vi "Finish.vi"(8 "error in (no error)":errorcluster, 11 "Dev Grabber in":refnum<class "Dev Grabber.lvclass">) -> (0 "error out":errorcluster, 3 "Dev Grabber out":refnum<class "Dev Grabber.lvclass">)   [LabVIEW 2014, in "Dev Grabber.lvlib" / "Dev Grabber.lvclass"]
uses:
  Dev Grabber.lvclass
  Dev Grabber.lvclass/Dev Grabber.ctl
  Robot/Grabber/Grabber Class/Grabber.lvclass
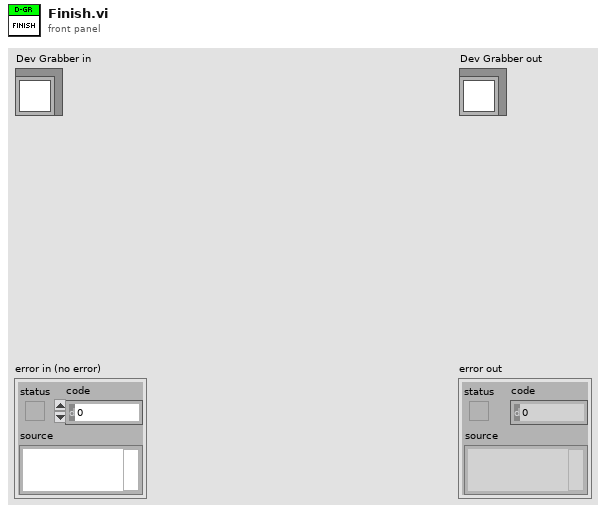
[diagram p1: front panel]
types:
  T1 = typedef "WPI_SolenoidDevRef.ctl" = cluster{"DevStatus":errorcluster, "Pneumatics Control Module":u8, "Forward Solenoid Channel":T2, "Reverse Solenoid Channel":T2}
  T2 = typedef "WPI_SolenoidChannel.ctl" = enum8{"Solenoid 0", "Solenoid 1", "Solenoid 2", "Solenoid 3", "Solenoid 4", "Solenoid 5", "Solenoid 6", "Solenoid 7", "Invalid"}
  T3 = typedef "WPI_MotorControlDeviceRef.ctl" = cluster{"DeviceStatus":errorcluster, "Type":T4, "PWM":cluster{"Controller":T5, "PWM Channel":T6, "DeadBand":T7}, "CAN":cluster{"Device Number":u8, "Control Mode":T8, "Semaphore":T9, "Max Vout":dbl, "TalonSRX Control Mode":T10}, "Invert":bool, "TransformRef":T11, "InvTransformRef":T11}
  T4 = typedef "WPI_MotorControlType.ctl" = enum16{"PWM", "CAN", "CANTalonSRX"}
  T5 = typedef "FPGA_TypedefDigitalModule.ctl" = enum16{"Controller 1"}
  T6 = typedef "FPGA_DIOPWMChannel.ctl" = enum8{"PWM 0", "PWM 1", "PWM 2", "PWM 3", "PWM 4", "PWM 5", "PWM 6", "PWM 7", "PWM 8", "PWM 9", "PWM MXP 0", "PWM MXP 1", "PWM MXP 2", "PWM MXP 3", "PWM MXP 4", "PWM MXP 5", "PWM MXP 6", "PWM MXP 7", "PWM MXP 8", "PWM MXP 9", "Invalid"}
  T7 = typedef "WPI_PWMDeadband.ctl" = cluster{"Name":string, "maxPositivePwm":i32, "minPositivePwm":i32, "centerPwm":i32, "maxNegativePwm":i32, "minNegativePwm":i32, "angularRange":u16}
  T8 = typedef "WPI_CANJaguar_ControlMode.ctl" = enum8{"Percent VBus", "Current", "Speed", "Position", "Voltage"}
  T9 = typedef "Semaphore RefNum" = refnum<k1>
  T10 = typedef "WPI_CANTalonSRX_APIControlMode.ctl" = enum8{"Percent VBus", "Speed", "Position", "Slave", "Unchanged / Invalid"}
  T11 = typedef "WPI_PWMTransform_ConPane.ctl" = refnum<vi>
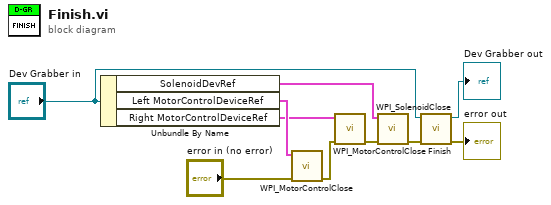
[diagram p0: block diagram]
diagram:
  n1 = Unbundle By Name("Dev Grabber in") -> ("SolenoidDevRef"=w7:T1, "Left MotorControlDeviceRef"=w2:T3, "Right MotorControlDeviceRef"=w1:T3)
  n2 = call <vilib>:"WPI_MotorControlClose.vi"("error in (no error)"="error in (no error)", "MotorControlDevRef"=w2) -> ("error out"=w4:errorcluster)  [unwired: 9 in]
  n3 = call <vilib>:"WPI_MotorControlClose.vi"("error in (no error)"=w4, "MotorControlDevRef"=w1) -> ("error out"=w3:errorcluster)  [unwired: 9 in]
  n4 = call <vilib>:"WPI_SolenoidClose.vi"("error in (no error)"=w3, "SolenoidDevRef"=w7) -> ("error out"=w6:errorcluster)  [unwired: 9 in]
  n5 = call-parent "Finish.vi"("error in (no error)"=w6, "System Actor in"="Dev Grabber in") -> ("error out"=→"error out":errorcluster, "System Actor out"=→"Dev Grabber out":refnum<class "Dev Grabber.lvclass">)  [unwired: 8 in]
